vi "SUB-Cal Table 피팅 데이터 변환-다항식 파라미터 계산 .vi"(6 "Index":u8 max=19 step=1, 8 "Page":u8=1 max=1 step=1, 9 "배열-센서 전압(V)":dbl[](array[numeric])=[3.71489239, 3.68351507, 3.58652544, 3.48851752, 3.3912003, 3.29144764, 3.19365191, 3.09626293, 2.99890614, 2.90132809, 2.8021009, 2.70419431, 2.60852098, 2.51315856, 2.41333866, 2.31576657, 2.21826339, 2.11889887, 2.02145934, 1.92394173, 1.82836294, 1.73020589, 1.63263667, 1.53490806, 1.43661809, 1.33888328, 1.24262989, 1.14526045, 1.04808402], 10 "배열-설정압력(psi)":dbl[](array[numeric])=[1.0, 1.5, 2.0, 2.5, 3.0, 3.5, 4.0, 4.5, 5.0, 5.5, 6.0, 6.5, 7.0, 7.5, 8.0, 8.5, 9.0, 9.5, 10.0, 10.5, 11.0, 11.5, 12.0, 12.5, 13.0, 13.5, 14.0, 14.5, 15.0], 11 "배열-온도(degC)":dbl[](array[numeric])=[27.010547637939453, 26.977344512939453, 27.014062881469727, 27.030858993530273, 27.033594131469727, 27.06640625, 27.046092987060547, 27.05078125, 27.064453125, 27.075780868530273]) -> (0 "residue":dbl=0.002310824325216588 caption="오차", 1 "온도, 다항식 계수":string="27.037, 1.920244E+1, -2.635180E+0, -1.882709E+0, 5.985099E-1, -6.784961E-2", 2 "문자열(Hex)":string="Page1 Index00: 41D84BC3, 41999E9B, C028A6CB, BFF0FC9D, 3F1937F2, BD8AF4BD, ", 3 "Tx 문자열":string="CALFLASHWR 9348293 1 0  1104694211 1100586651 3223889611 3220241565 1058617330 3180000445", 4 "그래프 이미지":T1={"image type"=0, "image depth"=24, "image"=array[1505520 elements], "mask"=[], "colors"=[], "Rectangle"={"left"=0, "top"=0, "right"=984, "bottom"=510}} caption="이미지 데이터")   [LabVIEW 2015]
uses:
  <vilib>/picture/picture.llb/imagedata.ctl
  <vilib>/Analysis/6fits.llb/Curve Fitting Criteria.ctl
  <vilib>/Analysis/6fits.llb/General Linear Fit Algorithm.ctl
  <vilib>/Analysis/baseanly.llb/Mean (DBL).vi
  <vilib>/Analysis/NI_AALPro.lvlib
  <vilib>/Analysis/NI_AALBase.lvlib
panel:
  out "온도 평균값":dbl=27.036992263793945 format="%0.2f"
  out "Best Polynomial Fit":dbl[](array[numeric])=[1.1926335154457703, 1.3725001978535865, 1.9189366148741627, 2.4581177214027097, 2.982585490724041, 3.5108348310135495, 4.02129468078433, 4.5239036021057615, 5.022048011274063, 5.518283237374725, 6.020943334179397, 6.515972422097601, 6.999614352605217, 7.482235977552367, 7.988551480173518, 8.484981278703604, 8.982800805083706, 9.4920093778735, 9.993145378642465, 10.496255413828207, 10.990551446980305, 11.498911061314613, 12.004315274279493, 12.509837917551462, 13.01659604036866, 13.517734002914906, 14.007377948157911, 14.497400291829074, 14.97962829301112] caption="최적 다항식 피팅"
  out "다항식 계수":dbl[](array[numeric])=[19.202444265309808, -2.635180167080928, -1.8827091470643729, 0.598509903050085, -0.06784961331388688] format="%#_7g"
  out "압력 vs 센서 전압 그래프":T2(graph)=[{"배열-설정압력(psi)"=[1.0, 1.5, 2.0, 2.5, 3.0, 3.5, 4.0, 4.5, 5.0, 5.5, 6.0, 6.5, 7.0, 7.5, 8.0, 8.5, 9.0, 9.5, 10.0, 10.5, 11.0, 11.5, 12.0, 12.5, 13.0, 13.5, 14.0, 14.5, 15.0], "Best Polynomial Fit"=[3.71489239, 3.68351507, 3.58652544, 3.48851752, 3.3912003, 3.29144764, 3.19365191, 3.09626293, 2.99890614, 2.90132809, 2.8021009, 2.70419431, 2.60852098, 2.51315856, 2.41333866, 2.31576657, 2.21826339, 2.11889887, 2.02145934, 1.92394173, 1.82836294, 1.73020589, 1.63263667, 1.53490806, 1.43661809, 1.33888328, 1.24262989, 1.14526045, 1.04808402]}, {"배열-설정압력(psi)"=[1.1926335154457703, 1.3725001978535865, 1.9189366148741627, 2.4581177214027097, 2.982585490724041, 3.5108348310135495, 4.02129468078433, 4.5239036021057615, 5.022048011274063, 5.518283237374725, 6.020943334179397, 6.515972422097601, 6.999614352605217, 7.482235977552367, 7.988551480173518, 8.484981278703604, 8.982800805083706, 9.4920093778735, 9.993145378642465, 10.496255413828207, 10.990551446980305, 11.498911061314613, 12.004315274279493, 12.509837917551462, 13.01659604036866, 13.517734002914906, 14.007377948157911, 14.497400291829074, 14.97962829301112], "Best Polynomial Fit"=[3.71489239, 3.68351507, 3.58652544, 3.48851752, 3.3912003, 3.29144764, 3.19365191, 3.09626293, 2.99890614, 2.90132809, 2.8021009, 2.70419431, 2.60852098, 2.51315856, 2.41333866, 2.31576657, 2.21826339, 2.11889887, 2.02145934, 1.92394173, 1.82836294, 1.73020589, 1.63263667, 1.53490806, 1.43661809, 1.33888328, 1.24262989, 1.14526045, 1.04808402]}]
  # "피팅 파라미터 생성\n>> 측정된 센서 전압과 압력 데이터를 기반으로 캘 테이블 관련 전송 명령서 생성"
  # "0 : APS\n1 : DPS"
  # "0~19"
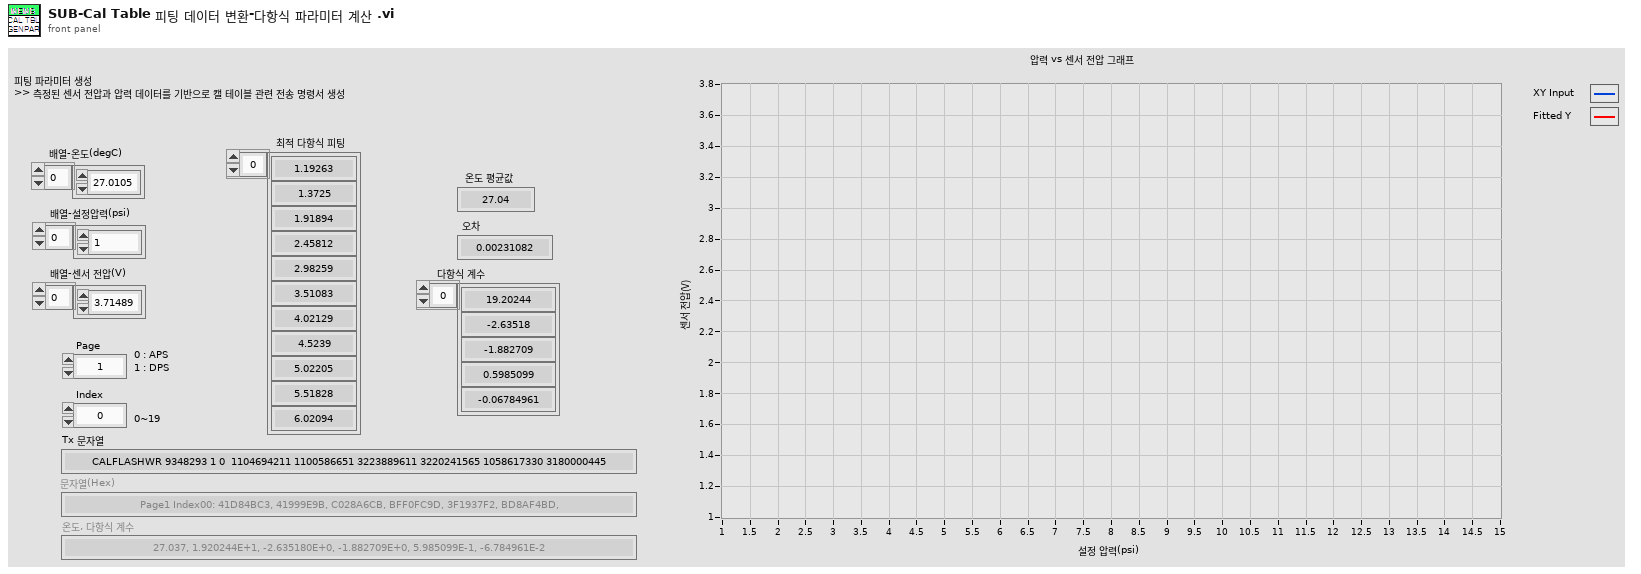
[diagram p1: front panel]
types:
  T1 = typedef "imagedata.ctl" = cluster{"image type":i32, "image depth":i32, "image":u8[], "mask":u8[], "colors":u32[], "Rectangle":cluster{"left":i16, "top":i16, "right":i16, "bottom":i16}}
  T2 = cluster{"배열-설정압력(psi)":dbl[], "Best Polynomial Fit":dbl[]}[]
  T3 = typedef "NI_AALPro.lvlib/General Linear Fit Algorithm.ctl" = u16
  T4 = typedef "NI_AALPro.lvlib/Curve Fitting Criteria.ctl" = u16
  T5 = cluster{"배열-설정압력(psi)":dbl[], "배열-센서 전압(V)":dbl[]}
  T6 = cluster{"Best Polynomial Fit":dbl[], "배열-센서 전압(V)":dbl[]}
  T7 = cluster{"Best Polynomial Fit":dbl[], "배열-센서 전압(V)":dbl[]}[]
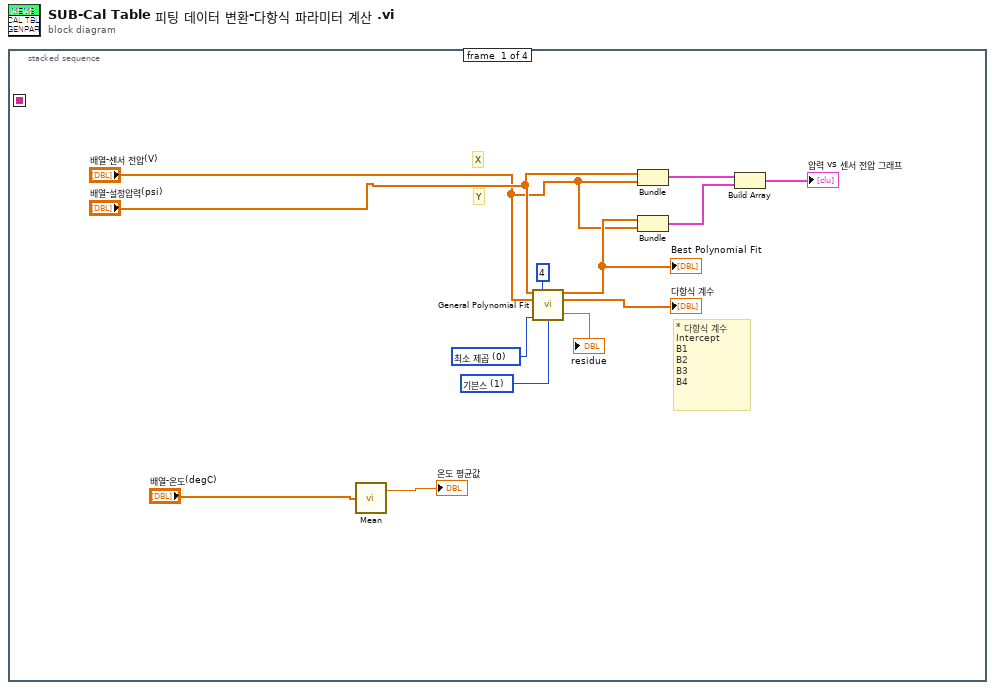
[diagram p0: block diagram]
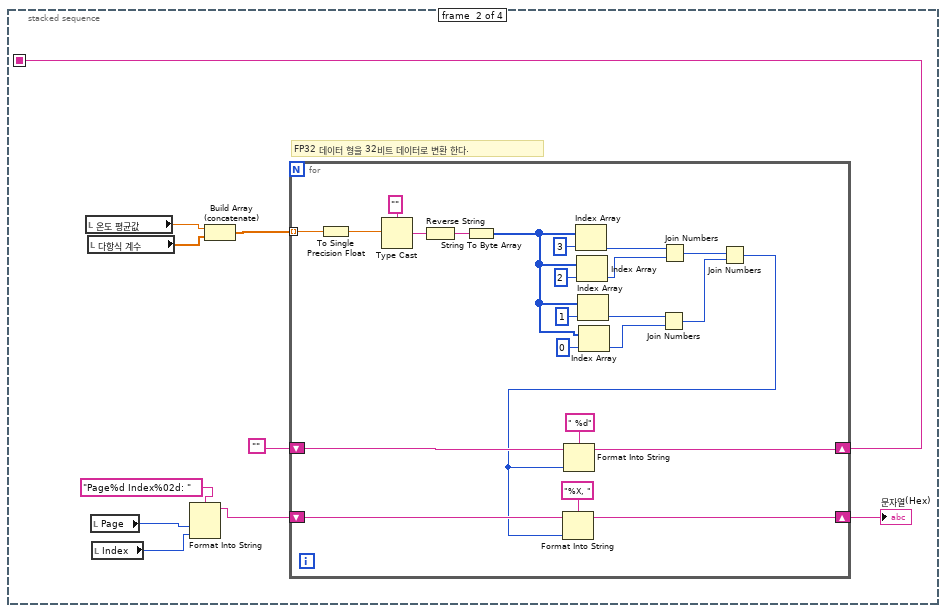
[diagram p2: hidden frame]
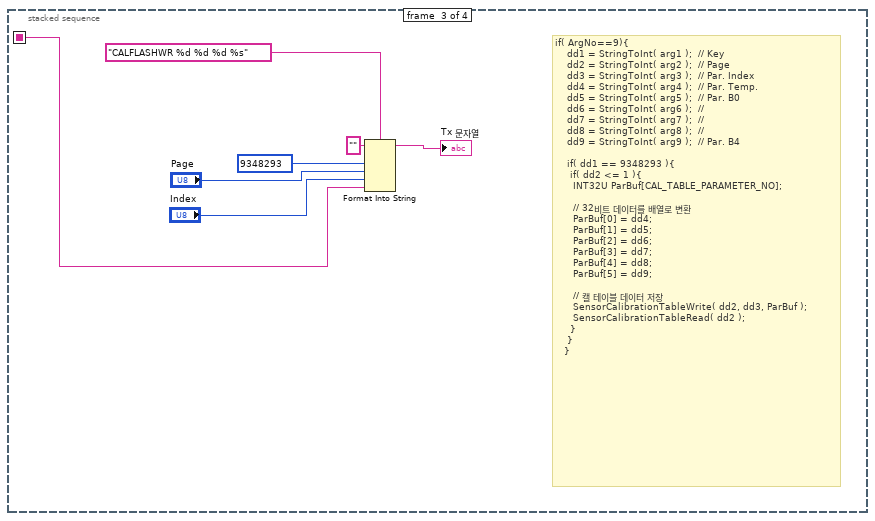
[diagram p3: hidden frame]
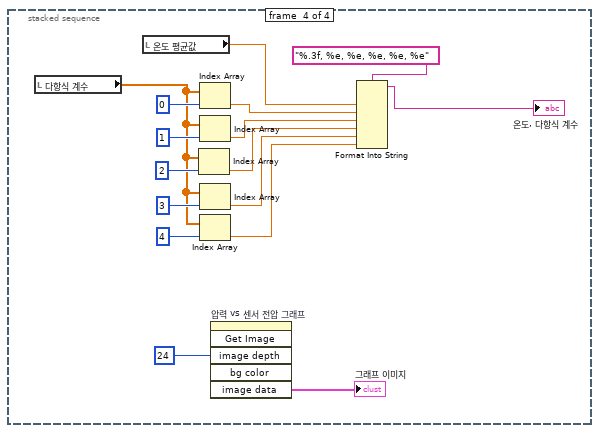
[diagram p4: hidden frame]
diagram:
  n1 = stacked-sequence {
    seq-local: [_ w20 _ _] -> [_ _ w47 _]
    frame #0 {
      w5 = T3 1 items=["SVD", "기븐스", "기븐스2", "하우스홀더", "LU 분해", "콜레스키", "계수가 부족한 H를 위한 SVD"] ("algorithm")
      w13 = T4 0 items=["최소 제곱", "최소 절대 오차", "바이스퀘어(Bisquare)"] ("method")
      # "Y"
      # "X"
      # "* 다항식 계수\nIntercept\nB1\nB2\nB3\nB4"
      n2 = call-poly <vilib>:"Mean.vi"("X"="배열-온도(degC)") -> ("mean"=→"온도 평균값":dbl)  [unwired: 1 out]
      n3 = call <vilib>:"General Polynomial Fit.vi"("Y"="배열-설정압력(psi)", "polynomial order"=4, "X"="배열-센서 전압(V)", "method"=w13, "algorithm"=w5) -> ("Best Polynomial Fit"=w2:dbl[], "Polynomial Coefficients"=→"다항식 계수":dbl[], "residue"=→"residue":dbl)  [unwired: 7 in, 1 out]
      "Best Polynomial Fit" <- w2
      n4 = Bundle("배열-설정압력(psi)"="배열-설정압력(psi)", "배열-센서 전압(V)"="배열-센서 전압(V)") -> (w10:T5)  [unwired: 1 in]
      n5 = Bundle("Best Polynomial Fit"=w2, "배열-센서 전압(V)"="배열-센서 전압(V)") -> (w9:T6)  [unwired: 1 in]
      n6 = Build Array(w10, w9) -> (→"압력 vs 센서 전압 그래프":T7)
    }
    frame #1 {
      # "FP32 데이터 형을 32비트 데이터로 변환 한다."
      n7 = local read "온도 평균값"() -> (w23:dbl)
      n8 = local read "다항식 계수"() -> (w22:dbl[])
      n9 = local read "Page"() -> (w17:u8)
      n10 = local read "Index"() -> (w16:u8)
      n11 = Format Into String(format string="Page%d Index%02d: " ("포맷 문자열"), w17, w16) -> (resulting string=w14:string)  [unwired: 2 in, 1 out]
      n12 = Build Array (concatenate)(w23, w22) -> (w21:dbl[])
      n13 = for {
        tunnel: w21 -> [w29] mode=indexing
        shift-right: [w30] -> w20
        shift-left: "" -> [w32]
        shift-right: [w26] -> w18
        shift-left: w14 -> [w27]
        n14 = To Single Precision Float(number=w29) -> (single precision float=w25:sgl)
        n15 = Type Cast(type="" ("타입"), x=w25) -> (*(type *) &x=w46:string)
        n16 = Reverse String(1:w46) -> (0:w45:string)
        n17 = String To Byte Array(string=w45) -> (unsigned byte array=w40:u8[])
        n18 = Index Array(array=w40, index=3 ("인덱스")) -> (element=w39:u8)
        n19 = Index Array(array=w40, index=2 ("인덱스")) -> (element=w38:u8)
        n20 = Index Array(array=w40, index=1 ("인덱스")) -> (element=w37:u8)
        n21 = Index Array(array=w40, index=0 ("인덱스")) -> (element=w36:u8)
        n22 = Join Numbers(hi=w37, lo=w36) -> ((hi.lo)=w34:u16)
        n23 = Join Numbers(hi=w39, lo=w38) -> ((hi.lo)=w35:u16)
        n24 = Join Numbers(hi=w35, lo=w34) -> ((hi.lo)=w24:u32)
        n25 = Format Into String(format string="%X, " ("포맷 문자열"), initial string=w27, w24) -> (resulting string=w26:string)  [unwired: 1 in, 1 out]
        n26 = Format Into String(format string=" %d" ("포맷 문자열"), initial string=w32, w24) -> (resulting string=w30:string)  [unwired: 1 in, 1 out]
      }
      "문자열(Hex)" <- w18
    }
    frame #2 {
      # "if( ArgNo==9){\n\t\t\t\tdd1 = StringToInt( arg1 );\t\t// Key\n\t\t\t\tdd2 = StringToInt( arg2 );\t\t// Page\n\t\t\t\tdd3 = StringToInt( arg3 );\t\t// Par. Index\n\t\t\t\tdd4 = StringToInt( arg4 );\t\t// Par. Temp.\n\t\t\t\tdd5 = StringToInt( arg5 );\t\t// Par. B0\n\t\t\t\tdd6 = StringToInt( arg6 );\t\t// \n\t\t\t\tdd7 = StringToInt( arg7 );\t\t// \n\t\t\t\tdd8 = StringToInt( arg8 );\t\t// \n\t\t\t\tdd9 = StringToInt( arg9 );\t\t// Par. B4\n\n\t\t\t\tif( dd1 == 9348293 ){\n\t\t\t\t\tif( dd2 <= 1 ){\n\t\t\t\t\t\tINT32U ParBuf[CAL_TABLE_PARAMETER_NO];\n\n\t\t\t\t\t\t// 32비트 데이터를 배열로 변환\n\t\t\t\t\t\tParBuf[0] = dd4;\n\t\t\t\t\t\tParBuf[1] = dd5;\n\t\t\t\t\t\tParBuf[2] = dd6;\n\t\t\t\t\t\tParBuf[3] = dd7;\n\t\t\t\t\t\tParBuf[4] = dd8;\n\t\t\t\t\t\tParBuf[5] = dd9;\n\n\t\t\t\t\t\t// 캘 테이블 데이터 저장\n\t\t\t\t\t\tSensorCalibrationTableWrite( dd2, dd3, ParBuf );\n\t\t\t\t\t\tSensorCalibrationTableRead( dd2 );\n\t\t\t\t\t}\n\t\t\t\t}\n\t\t\t}"
      n27 = Format Into String(format string="CALFLASHWR %d %d %d %s" ("포맷 문자열"), initial string="" ("초기 문자열"), 9348293, "Page", "Index", w47) -> (resulting string=→"Tx 문자열":string)  [unwired: 1 in, 1 out]
    }
    frame #3 {
      n28 = local read "다항식 계수"() -> (w62:dbl[])
      n29 = local read "온도 평균값"() -> (w54:dbl)
      n30 = Index Array(array=w62, index=2 ("인덱스")) -> (element=w60:dbl)
      n31 = Index Array(array=w62, index=0 ("인덱스")) -> (element=w55:dbl)
      n32 = Index Array(array=w62, index=1 ("인덱스")) -> (element=w61:dbl)
      n33 = Index Array(array=w62, index=3 ("인덱스")) -> (element=w59:dbl)
      n34 = Index Array(array=w62, index=4 ("인덱스")) -> (element=w58:dbl)
      n35 = invoke on="압력 vs 센서 전압 그래프" class="XYGraph (엄격한)" method="Get Image"("image depth"=24 ("이미지 농도")) -> ("image data"=→"그래프 이미지":T1)  [unwired: 5 in, 5 out]
      n36 = Format Into String(format string="%.3f, %e, %e, %e, %e, %e" ("텍스트 입력"), w54, w55, w61, w60, w59, w58) -> (resulting string=→"온도, 다항식 계수":string)  [unwired: 2 in, 1 out]
    }
  }
